vi "DiffDrivePoseEst2_ResetPosition.vi"(6 "Pose":T7={"TRANSLATION"={"X"=0.0, "Y"=0.0}, "ROTATION"={"VALUE"=0.0, "COS"=1.0, "SIN"=0.0}} {"ROTATION"."SIN" format="%13.4f"; "ROTATION"."COS" format="%13.4f"; "ROTATION"."VALUE" format="%13.4f"; "TRANSLATION"."Y" format="%14.3f"; "TRANSLATION"."X" format="%14.3f"}, 8 "RightDistance_M":dbl, 9 "LeftDistance_M":dbl, 10 "Gyro":T1={"VALUE"=0.0, "COS"=1.0, "SIN"=0.0} {"SIN" format="%13.4f"; "COS" format="%13.4f"; "VALUE" format="%13.4f"}, 11 "in DiffDrivePoseEst2":T2={"M_Vision_K"=[], "m_nominal_dT"=0.0, "m_PrevTime_Sec"=0.0, "Pose_Buffer"={"TimeStamps"=[], "DataArray"=[], "Min_TimeStamp"=0.0, "Max_TimeStamp"=0.0, "ItemCount"=0, "MaxBufferTime"=0.0}, "Diff_Drive_Kinematics"={"TrackWidth_Meters"=0.0}, "Diff_Drive_Odom_2"={"M_POSE_Meters"={"TRANSLATION"={"X"=0.0, "Y"=0.0}, "ROTATION"={"VALUE"=0.0, "COS"=1.0, "SIN"=0.0}}, "M_GyroOffset"={"VALUE"=0.0, "COS"=1.0, "SIN"=0.0}, "M_PrevAngle"={"VALUE"=0.0, "COS"=1.0, "SIN"=0.0}, "M_PrevLeftDist_M"=0.0, "M_PrevRightDist_M"=0.0, "M_InitLeftDist_M"=0.0, "M_InitRightDist_M"=0.0}, "M_Q"=[[0.0], [0.0], [0.0]]} {"Diff_Drive_Odom_2"."M_PrevAngle"."SIN" format="%13.4f"; "Diff_Drive_Odom_2"."M_PrevAngle"."COS" format="%13.4f"; "Diff_Drive_Odom_2"."M_PrevAngle"."VALUE" format="%13.4f"; "Diff_Drive_Odom_2"."M_GyroOffset"."SIN" format="%13.4f"; "Diff_Drive_Odom_2"."M_GyroOffset"."COS" format="%13.4f"; "Diff_Drive_Odom_2"."M_GyroOffset"."VALUE" format="%13.4f"; "Diff_Drive_Odom_2"."M_POSE_Meters"."ROTATION"."SIN" format="%13.4f"; "Diff_Drive_Odom_2"."M_POSE_Meters"."ROTATION"."COS" format="%13.4f"; "Diff_Drive_Odom_2"."M_POSE_Meters"."ROTATION"."VALUE" format="%13.4f"; "Diff_Drive_Odom_2"."M_POSE_Meters"."TRANSLATION"."Y" format="%14.3f"; "Diff_Drive_Odom_2"."M_POSE_Meters"."TRANSLATION"."X" format="%14.3f"; "Diff_Drive_Kinematics"."TrackWidth_Meters" format="%20.4f"}) -> (3 "Out DiffDrivePoseEst2":T2={"M_Vision_K"=[], "m_nominal_dT"=0.0, "m_PrevTime_Sec"=0.0, "Pose_Buffer"={"TimeStamps"=[], "DataArray"=[], "Min_TimeStamp"=0.0, "Max_TimeStamp"=0.0, "ItemCount"=0, "MaxBufferTime"=0.0}, "Diff_Drive_Kinematics"={"TrackWidth_Meters"=0.0}, "Diff_Drive_Odom_2"={"M_POSE_Meters"={"TRANSLATION"={"X"=0.0, "Y"=0.0}, "ROTATION"={"VALUE"=0.0, "COS"=1.0, "SIN"=0.0}}, "M_GyroOffset"={"VALUE"=0.0, "COS"=1.0, "SIN"=0.0}, "M_PrevAngle"={"VALUE"=0.0, "COS"=1.0, "SIN"=0.0}, "M_PrevLeftDist_M"=0.0, "M_PrevRightDist_M"=0.0, "M_InitLeftDist_M"=0.0, "M_InitRightDist_M"=0.0}, "M_Q"=[[0.0], [0.0], [0.0]]} {"Diff_Drive_Odom_2"."M_PrevAngle"."SIN" format="%13.4f"; "Diff_Drive_Odom_2"."M_PrevAngle"."COS" format="%13.4f"; "Diff_Drive_Odom_2"."M_PrevAngle"."VALUE" format="%13.4f"; "Diff_Drive_Odom_2"."M_GyroOffset"."SIN" format="%13.4f"; "Diff_Drive_Odom_2"."M_GyroOffset"."COS" format="%13.4f"; "Diff_Drive_Odom_2"."M_GyroOffset"."VALUE" format="%13.4f"; "Diff_Drive_Odom_2"."M_POSE_Meters"."ROTATION"."SIN" format="%13.4f"; "Diff_Drive_Odom_2"."M_POSE_Meters"."ROTATION"."COS" format="%13.4f"; "Diff_Drive_Odom_2"."M_POSE_Meters"."ROTATION"."VALUE" format="%13.4f"; "Diff_Drive_Odom_2"."M_POSE_Meters"."TRANSLATION"."Y" format="%14.3f"; "Diff_Drive_Odom_2"."M_POSE_Meters"."TRANSLATION"."X" format="%14.3f"; "Diff_Drive_Kinematics"."TrackWidth_Meters" format="%20.4f"})   [LabVIEW 2019, in "Trajectory_Library.lvlib"]
doc: "Resets the robot's position on the field.\n \nThe gyroscope angle does not need to be reset here on the user's robot code. The library automatically takes care of offsetting the gyro angle.\n \nInputs:\n - inDiffDrvPoseEst2 -- DifDrvPoseEst2 -- Data cluster\n - gyroAngle -- Rotation2d -- The angle reported by the gyroscope.\n - leftPositionMeters -- double -- The distance traveled by the left encoder.\n - rightPositionMeters -- double -- The distance traveled by the right encoder.\n - poseMeters -- Pose2d -- The position on the field that your robot is at.\n\nOutputs:\n - outDiffDrvPoseEst2 -- DifDrvPoseEst2 -- Updated data cluster"
uses:
  Trajectory_Library.lvlib
  TypeDef/DIFF_DRIVE_POSE_EST2.ctl
  <vilib>/Analysis/Matrix/Datatypes/RealMatrix.ctl
  TypeDef/TIME_INTERPOLATABLE_VARIANT.ctl
  TypeDef/DIFF_DRIVE_KINEMATICS.ctl
  TypeDef/DIFF_DRIVE_ODOM2.ctl
  TypeDef/POSE2D.ctl
  TypeDef/TRANSLATION2D.ctl
  TypeDef/ROTATION2D.ctl
  Pose2d_getRotation.vi
  Rotation2d_Minus.vi
  Rotation2d_UnaryMinus.vi
  Rotation2d_RotateBy.vi
  Rotation2d_CreateAngle.vi
  Rotation2d_CreateXY.vi
  Util_CalcDist.vi
  <vilib>/Analysis/Matrix/NI_Matrix.lvlib
panel:
  # "<3, 1>"
  # "<3, 3>"
  # "<3, 1>"
  # "<3, 3>"
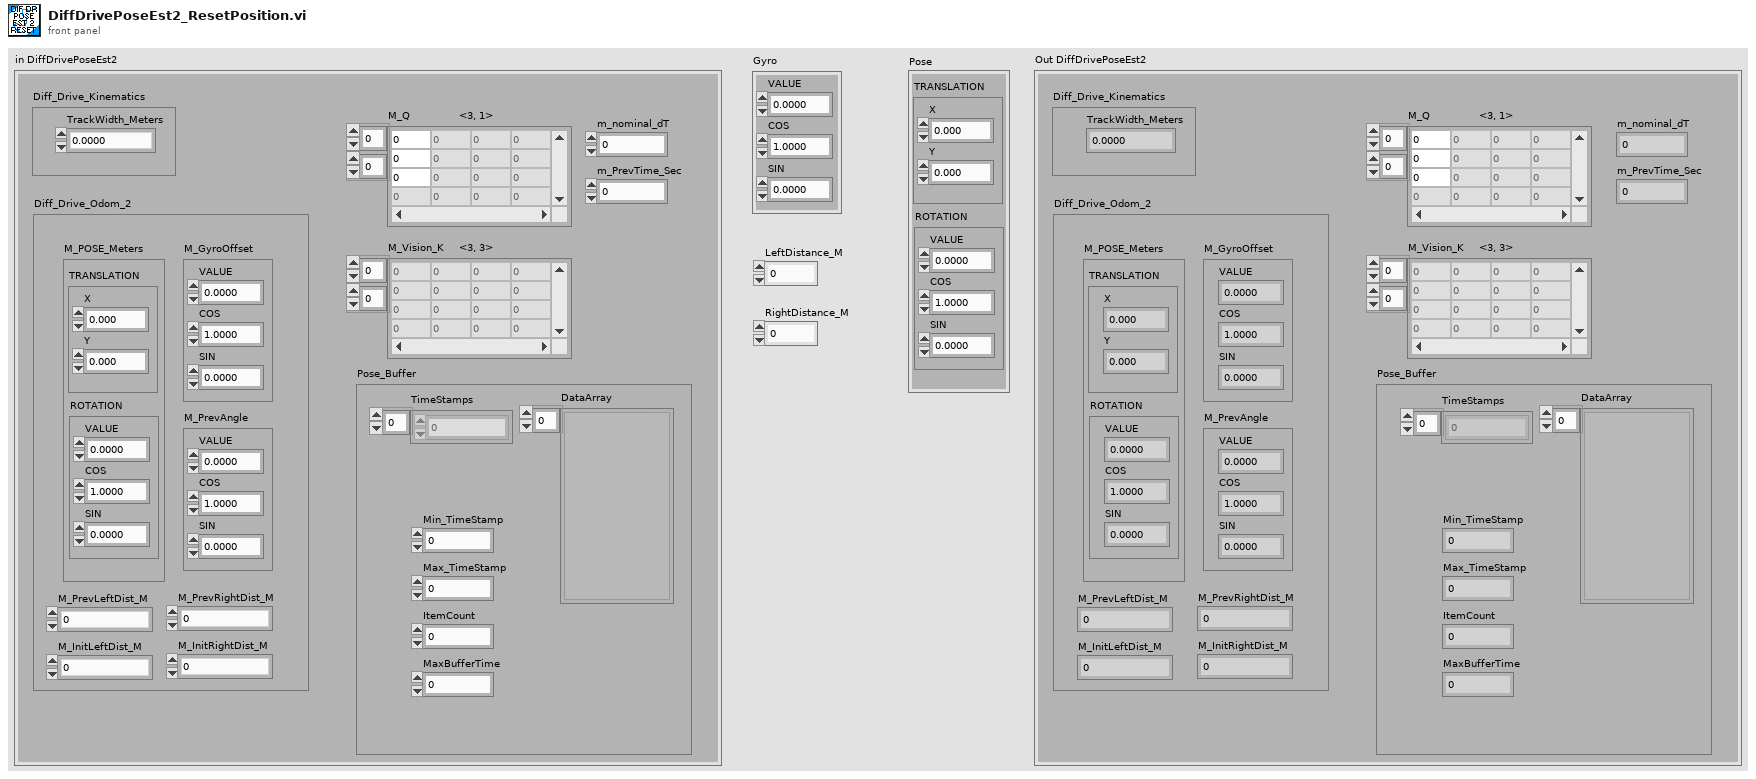
[diagram p1: front panel]
types:
  T1 = typedef "Trajectory_Library.lvlib/ROTATION2D.ctl" = cluster{"VALUE":dbl, "COS":dbl, "SIN":dbl}
  T2 = typedef "Trajectory_Library.lvlib/DIFF_DRIVE_POSE_EST2.ctl" = cluster{"M_Vision_K":T3, "m_nominal_dT":dbl, "m_PrevTime_Sec":dbl, "Pose_Buffer":T4, "Diff_Drive_Kinematics":T5, "Diff_Drive_Odom_2":T6, "M_Q":T3}
  T3 = typedef "NI_Matrix.lvlib/RealMatrix.ctl" = dbl[][]
  T4 = typedef "Trajectory_Library.lvlib/TIME_INTERPOLATABLE_VARIANT.ctl" = cluster{"TimeStamps":dbl[], "DataArray":variant[], "Min_TimeStamp":dbl, "Max_TimeStamp":dbl, "ItemCount":i32, "MaxBufferTime":dbl}
  T5 = typedef "Trajectory_Library.lvlib/DIFF_DRIVE_KINEMATICS.ctl" = cluster{"TrackWidth_Meters":dbl}
  T6 = typedef "Trajectory_Library.lvlib/DIFF_DRIVE_ODOM2.ctl" = cluster{"M_POSE_Meters":T7, "M_GyroOffset":T1, "M_PrevAngle":T1, "M_PrevLeftDist_M":dbl, "M_PrevRightDist_M":dbl, "M_InitLeftDist_M":dbl, "M_InitRightDist_M":dbl}
  T7 = typedef "Trajectory_Library.lvlib/POSE2D.ctl" = cluster{"TRANSLATION":T8, "ROTATION":T1}
  T8 = typedef "Trajectory_Library.lvlib/TRANSLATION2D.ctl" = cluster{"X":dbl, "Y":dbl}
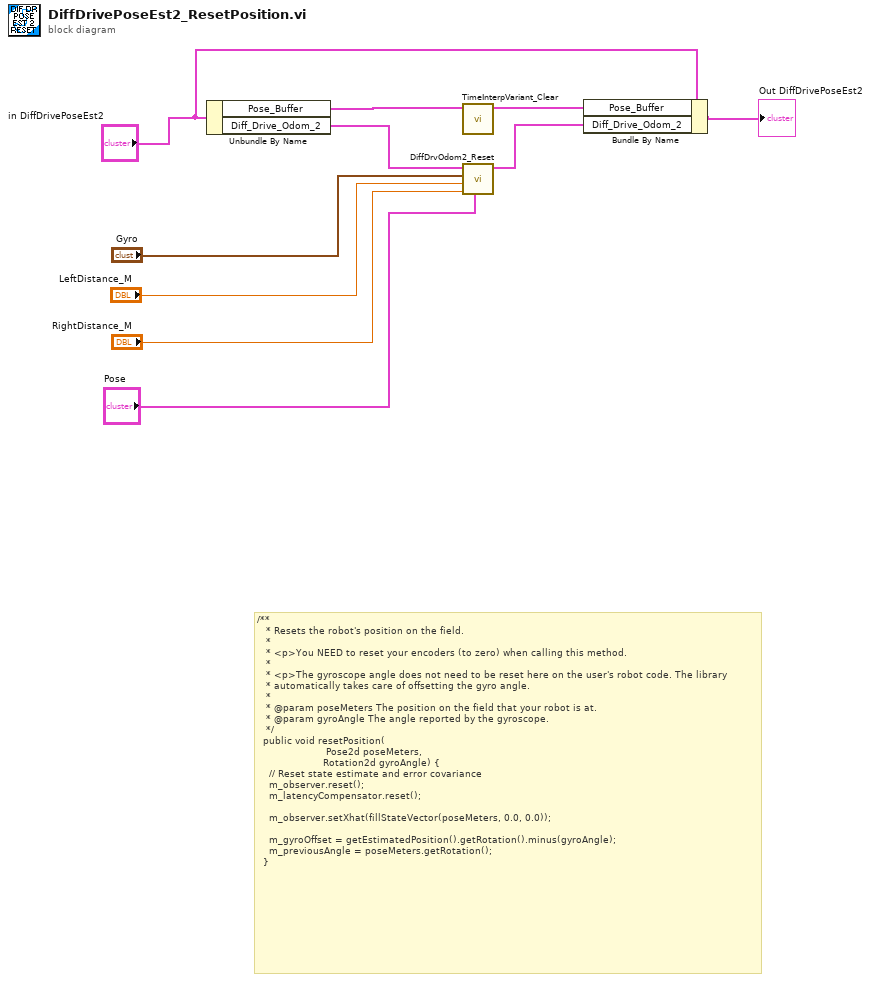
[diagram p0: block diagram]
diagram:
  # "/**\n   * Resets the robot's position on the field.\n   *\n   * <p>You NEED to reset your encoders (to zero) when calling this method.\n   *\n   * <p>The gyroscope angle does not need to be reset here on the user's robot code. The library\n   * automatically takes care of offsetting the gyro angle.\n   *\n   * @param poseMeters The position on the field that your robot is at.\n   * @param gyroAngle The angle reported by the gyroscope.\n   */\n  public void resetPosition(\n                       Pose2d poseMeters, \n                      Rotation2d gyroAngle) {\n    // Reset state estimate and error covariance\n    m_observer.reset();\n    m_latencyCompensator.reset();\n\n    m_observer.setXhat(fillStateVector(poseMeters, 0.0, 0.0));\n\n    m_gyroOffset = getEstimatedPosition().getRotation().minus(gyroAngle);\n    m_previousAngle = poseMeters.getRotation();\n  }"
  n1 = Unbundle By Name("in DiffDrivePoseEst2") -> ("Pose_Buffer"=w9:T4, "Diff_Drive_Odom_2"=w6:T6)
  n2 = call "TimeInterpVariant_Clear.vi"("in TimeInterpVariant"=w9) -> ("out TimeInterpVariant"=w8:T4)  [unwired: 10 in]
  n3 = call "DiffDrvOdom2_Reset.vi"("Pose Meters"="Pose", "Right Distance M"="RightDistance_M", "Left Distance M"="LeftDistance_M", "Gyro Reading"="Gyro", "In DIFF_DRIVE_ODOM"=w6) -> ("Out DIFF_DRIVE_ODOM"=w5:T6)  [unwired: 6 in]
  n4 = Bundle By Name(cluster="in DiffDrivePoseEst2", "Pose_Buffer"=w8, "Diff_Drive_Odom_2"=w5) -> (→"Out DiffDrivePoseEst2":T2)
